vi "Initialize AVI files.vi"(6 "Save AVI?":bool, 9 "Camera 2?":bool, 10 "AVI File Path 2":path, 11 "AVI File Path":path) -> (2 "AVI Refnum 2":T1, 3 "AVI Refnum 1":T1)   [LabVIEW 2018]
uses:
  <vilib>/vision/Avi.llb/IMAQ AVI2 Refnum.ctl
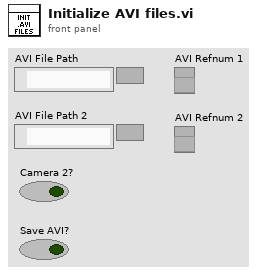
[diagram p1: front panel]
types:
  T1 = typedef "IMAQ AVI2 Refnum.ctl" = refnum<k20>
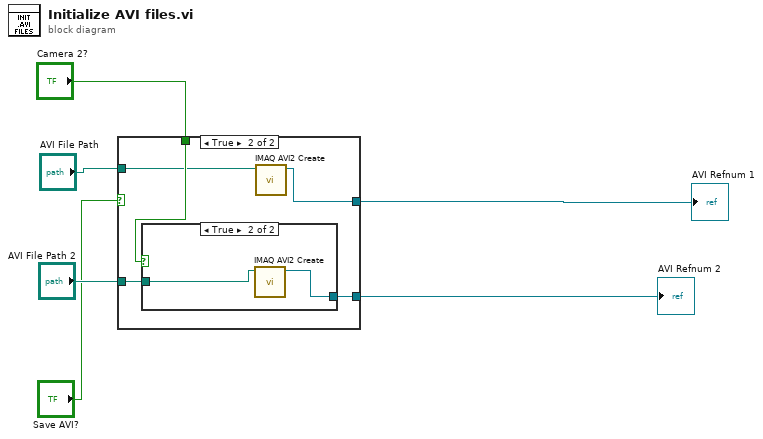
[diagram p0: block diagram]
diagram:
  n1 = case shown="True" "Save AVI?" {
    tunnel: [_ w11] -> w1
    tunnel: "Camera 2?" -> [_ w10]
    tunnel: [_ w9] -> w3
    tunnel: "AVI File Path 2" -> [_ w8]
    tunnel: "AVI File Path" -> [_ w7]
    frame False {
    }
    frame True {
      n2 = case shown="True" w10 {
        tunnel: [_ w13] -> w9
        tunnel: w8 -> [_ w12]
        frame False {
        }
        frame True {
          n3 = call "IMAQ AVI2 Create"("AVI Path"=w12) -> ("AVI Refnum"=w13:T1)  [unwired: 9 in, 1 out]
        }
      }
      n4 = call "IMAQ AVI2 Create"("AVI Path"=w7) -> ("AVI Refnum"=w11:T1)  [unwired: 9 in, 1 out]
    }
  }
  "AVI Refnum 2" <- w3
  "AVI Refnum 1" <- w1
